vi "ExposeMapperGetRawValueType.vi"(10 "Value":variant, 11 "Data Val Ref in":refnum<data-value>) -> (2 "IsNumeric":bool, 3 "MatlabType":T1)   [LabVIEW 2017]
uses:
  ExposeMapperDataTypeEnum.ctl
  <vilib>/Utility/Data Type/NI_Data Type.lvlib
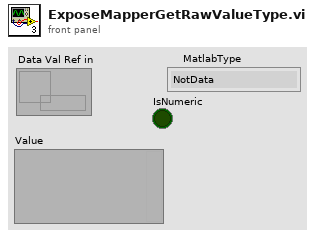
[diagram p1: front panel]
types:
  T1 = typedef "ExposeMapperDataTypeEnum.ctl" = enum16{"NotData", "int8", "byte", "int16", "uint16", "int32", "uint32", "int64", "uint64", "Single", "Double", "String", "Boolean", "Container"}
  T2 = typedef "NI_Data Type.lvlib/Data Type.ctl" = enum8{"Invalid Type", "Void", "I8", "I16", "I32", "I64", "U8", "U16", "U32", "U64", "Single Float", "Double Float", "Extended Float", "Single Complex", "Double Complex", "Extended Complex", "Enum U8", "Enum U16", "Enum U32", "Enum U64", "Single Float With Unit", "Double Float With Unit", "Extended Float With Unit", "Single Complex with Unit", "Double Complex with Unit", "Extended Complex with Unit", "Boolean", "String", "Path", "Picture", "Tag", "Array", "Cluster", "Variant", "LV Variant", "Waveform", "Timestamp", "Digital Waveform", "Digital Data", "ExpressData", "Refnum", "External Data", "VI", "Poly VI", "LabVIEW Class Instance", "Fixed Point"}
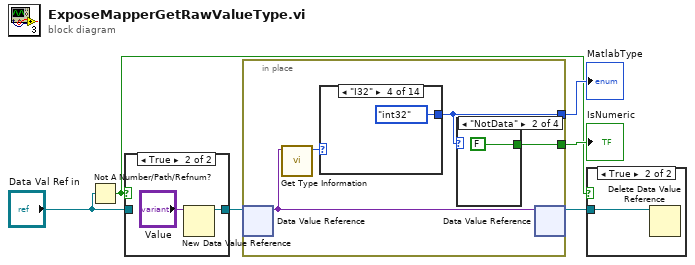
[diagram p0: block diagram]
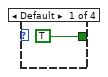
[diagram p4: hidden frame]
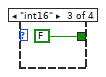
[diagram p5: hidden frame]
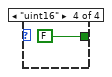
[diagram p6: hidden frame]
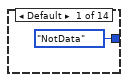
[diagram p7: hidden frame]
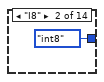
[diagram p8: hidden frame]
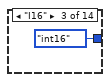
[diagram p9: hidden frame]
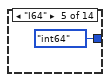
[diagram p10: hidden frame]
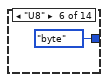
[diagram p11: hidden frame]
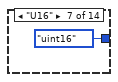
[diagram p12: hidden frame]
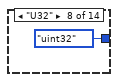
[diagram p13: hidden frame]
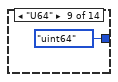
[diagram p14: hidden frame]
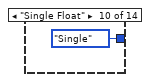
[diagram p15: hidden frame]
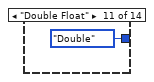
[diagram p16: hidden frame]
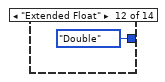
[diagram p17: hidden frame]
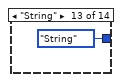
[diagram p18: hidden frame]
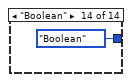
[diagram p19: hidden frame]
diagram:
  n1 = Not A Number/Path/Refnum?(number/path/refnum="Data Val Ref in") -> (NaN/Path/Refnum?=w2:bool)
  n2 = case shown="True" w2 {
    tunnel: "Data Val Ref in" -> [w7 _]
    tunnel: [w7 w8] -> w3
    frame False {
    }
    frame True {
      n3 = New Data Value Reference(data value="Value") -> (data value reference=w8:refnum<data-value>)  [unwired: 1 in, 1 out]
    }
  }
  n4 = in-place {
    in-place-border: [w12] -> w6
    in-place-border: [w11] -> w5
    n5 = in-place-dvr #1(w3) -> (w10:variant)  [unwired: 1 out]
    n6 = call <vilib>:"Get Type Information.vi"("Variant"=w10) -> ("Type"=w13:T2)  [unwired: 6 in, 4 out]
    n7 = case shown="\"I32\"" w13 {
      tunnel: [ExposeMapperDataTypeEnum."NotData" ("MatlabType") ExposeMapperDataTypeEnum."int8" ("MatlabType") ExposeMapperDataTypeEnum."int16" ("MatlabType") ExposeMapperDataTypeEnum."int32" ("MatlabType") ExposeMapperDataTypeEnum."int64" ("MatlabType") ExposeMapperDataTypeEnum."byte" ("MatlabType") ExposeMapperDataTypeEnum."uint16" ("MatlabType") ExposeMapperDataTypeEnum."uint32" ("MatlabType") ExposeMapperDataTypeEnum."uint64" ("MatlabType") ExposeMapperDataTypeEnum."Single" ("MatlabType") ExposeMapperDataTypeEnum."Double" ("MatlabType") ExposeMapperDataTypeEnum."Double" ("MatlabType") ExposeMapperDataTypeEnum."String" ("MatlabType") ExposeMapperDataTypeEnum."Boolean" ("MatlabType")] -> w11
      frame Default {
      }
      frame "I8" {
      }
      frame "I16" {
      }
      frame "I32" {
      }
      frame "I64" {
      }
      frame "U8" {
      }
      frame "U16" {
      }
      frame "U32" {
      }
      frame "U64" {
      }
      frame "Single Float" {
      }
      frame "Double Float" {
      }
      frame "Extended Float" {
      }
      frame "String" {
      }
      frame "Boolean" {
      }
    }
    n8 = case shown="\"NotData\"" w11 {
      tunnel: [TRUE FALSE FALSE FALSE] -> w12
      frame Default {
      }
      frame "NotData" {
      }
      frame "int16" {
      }
      frame "uint16" {
      }
    }
    n9 = in-place-dvr #1(w10) -> (w1:refnum<data-value>)  [unwired: 1 out]
  }
  "MatlabType" <- w5
  "IsNumeric" <- w6
  n10 = case shown="True" w2 {
    tunnel: w1 -> [_ w32]
    frame False {
    }
    frame True {
      n11 = Delete Data Value Reference(data value reference=w32) -> ()  [unwired: 1 in, 2 out]
    }
  }
